vi "Get Protocol Switch Threshold.vi"(8 "error in":errorcluster, 11 "Block Upload Initiate Transfer in":refnum<class "Block Upload Initiate Transfer.lvclass">) -> (0 "error out":errorcluster, 2 "Protocol Switch Threshold":u8, 3 "Block Upload Initiate Transfer out":refnum<class "Block Upload Initiate Transfer.lvclass">)   [LabVIEW 2020, in "CANopen.lvlib" / "SDO Manager.lvlib" / "Block Upload Initiate Transfer.lvclass"]
uses:
  Block Upload Initiate Transfer.lvclass
  Block Upload Initiate Transfer.lvclass/Block Upload Initiate Transfer.ctl
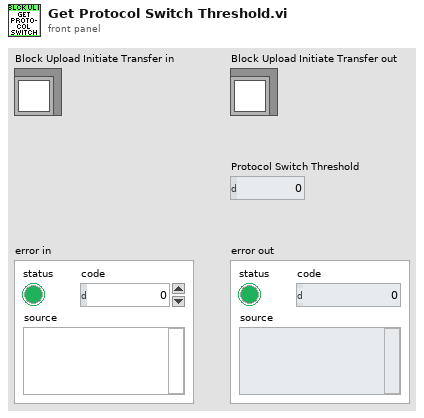
[diagram p1: front panel]
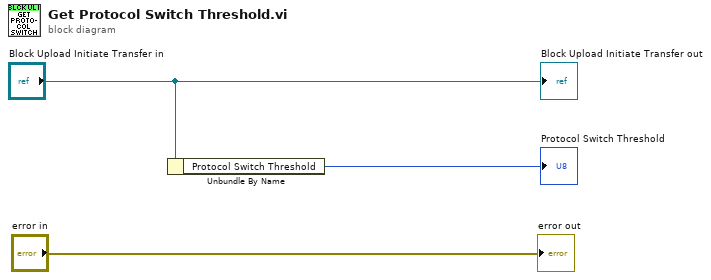
[diagram p0: block diagram]
diagram:
  n1 = Unbundle By Name("Block Upload Initiate Transfer in") -> ("Protocol Switch Threshold"=→"Protocol Switch Threshold":u8)
  "error out" <- "error in"
  "Block Upload Initiate Transfer out" <- "Block Upload Initiate Transfer in"
